vi "save.vi"(8 "error in (no error)":errorcluster, 10 "file refnum in":refnum<file>, 11 "RoiGeneric in":refnum<class "RoiGeneric.lvclass">) -> (0 "error out":errorcluster, 2 "file refnum out":refnum<file>, 3 "RoiGeneric out":refnum<class "RoiGeneric.lvclass">)   [LabVIEW 2010, in "RoiGeneric.lvclass"]
uses:
  RoiGeneric.lvclass
  xml_cluster.ctl
  attributes_cluster.ctl
  space_vector_cluster.ctl
  <vilib>/regexp/Match Regular Expression.xnode
  common/classes/Box/Box/Box.lvclass
  common/classes/SpaceVector/SpaceVector/SpaceVector.lvclass
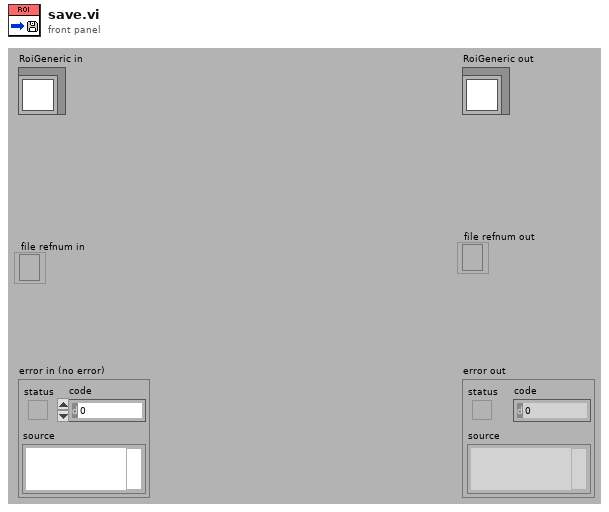
[diagram p1: front panel]
types:
  T1 = typedef "RoiGeneric.lvclass/xml_cluster.ctl" = cluster{"#attributes":T2, "center":T3, "dimensions":T3}
  T2 = typedef "RoiGeneric.lvclass/attributes_cluster.ctl" = cluster{"type":string, "ID":string}
  T3 = typedef "RoiGeneric.lvclass/space_vector_cluster.ctl" = cluster{"x":dbl[unit], "y":dbl[unit], "z":dbl[unit]}
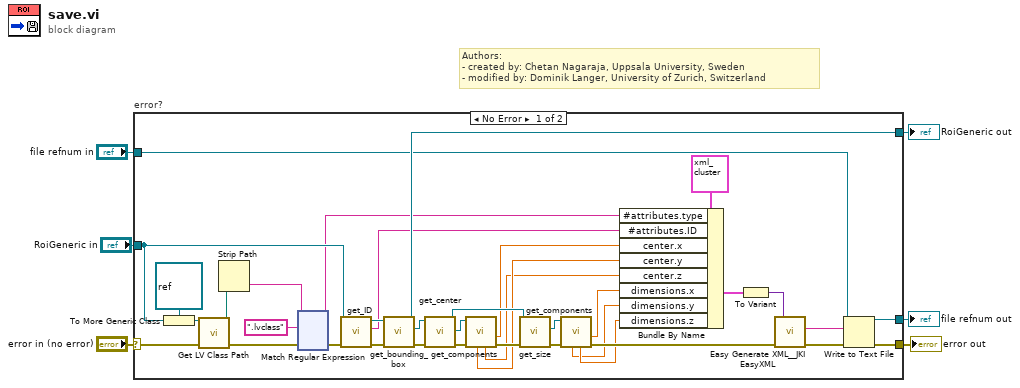
[diagram p0: block diagram]
diagram:
  # "Authors: \n- created by: Chetan Nagaraja, Uppsala University, Sweden\n- modified by: Dominik Langer, University of Zurich, Switzerland"
  n1 = case "error?" shown="No Error" "error in (no error)" {
    selector: "error in (no error)" -> [w16 w157]
    tunnel: [w21 w157] -> w5
    tunnel: [w39 w156] -> w3
    tunnel: "RoiGeneric in" -> [w14 w156]
    tunnel: "file refnum in" -> [w23 w155]
    tunnel: [w20 w155] -> w1
    frame No Error {
      n2 = To More Generic Class(target class=refnum<class> refnum ("LabVIEW Object"), reference=w14) -> (generic class reference=w13:refnum<class>)
      n3 = call <vilib>:"Get LV Class Path.vi"("error in (no error)"=w16, "object"=w13) -> ("error out"=w11:errorcluster, "class path"=w12:path)  [unwired: 8 in]
      n4 = Strip Path(path=w12) -> (name=w9:string)  [unwired: 1 out]
      n5 = xnode "Match Regular Expression"("input string"=w9, "regular expression"=".lvclass", "error in"=w11) -> ("before match"=w7:string, "error out"=w10:errorcluster)  [unwired: 3 in, 3 out]
      n6 = call-dynamic "get_ID.vi"("error in (no error)"=w10, "RoiGeneric in"=w14) -> ("error out"=w19:errorcluster, "ID"=w17:string, "RoiGeneric out"=w18:refnum<class "RoiGeneric.lvclass">)  [unwired: 7 in]
      n7 = call-dynamic "get_bounding_box.vi"("error in (no error)"=w19, "RoiGeneric in"=w18) -> ("error out"=w40:errorcluster, "Box.lvclass"=w38:refnum<class "Box.lvclass">, "RoiGeneric out"=w39:refnum<class "RoiGeneric.lvclass">)  [unwired: 7 in]
      n8 = call "get_center.vi"("error in (no error)"=w40, "Box in"=w38) -> ("error out"=w37:errorcluster, "center"=w35:refnum<class "SpaceVector.lvclass">, "Box out"=w32:refnum<class "Box.lvclass">)  [unwired: 7 in]
      n9 = call "get_components.vi"("error in (no error)"=w37, "SpaceVector in"=w35) -> ("error out"=w36:errorcluster, "x"=w30:dbl[unit], "z"=w28:dbl[unit], "y"=w29:dbl[unit])  [unwired: 4 in, 2 out]
      n10 = call "get_size.vi"("error in (no error)"=w36, "Box in"=w32) -> ("error out"=w34:errorcluster, "size"=w31:refnum<class "SpaceVector.lvclass">)  [unwired: 7 in, 1 out]
      n11 = call "get_components.vi"("error in (no error)"=w34, "SpaceVector in"=w31) -> ("error out"=w33:errorcluster, "x"=w27:dbl[unit], "z"=w26:dbl[unit], "y"=w25:dbl[unit])  [unwired: 4 in, 2 out]
      n12 = Bundle By Name(cluster=T1 {"#attributes"={"type"="ROI", "ID"=""}, "center"={"x"=0.0, "y"=0.0, "z"=0.0}, "dimensions"={"x"=0.0, "y"=0.0, "z"=0.0}} ("RoiGeneric"), "#attributes.type"=w7, "#attributes.ID"=w17, "center.x"=w30, "center.y"=w29, "center.z"=w28, "dimensions.x"=w27, "dimensions.y"=w25, "dimensions.z"=w26) -> (w41:T1)
      n13 = To Variant(anything=w41) -> (Variant=w42:variant)
      n14 = call <vilib>:"Easy Generate XML__JKI EasyXML.vi"("error in (no error)"=w33, "LabVIEW Data"=w42) -> ("error out"=w22:errorcluster, "XML String"=w24:string)  [unwired: 8 in]
      n15 = Write to Text File(file (use dialog)=w23, text=w24, error in=w22) -> (refnum out=w20:refnum<file>, error out=w21:errorcluster)  [unwired: 1 in, 1 out]
    }
    frame Error {
    }
  }
  "error out" <- w5
  "RoiGeneric out" <- w3
  "file refnum out" <- w1
